vi "DefinePosition.vi"(4 "error in (no error)":errorcluster, 6 "homePosition":i32, 7 "axis in":cluster{"keyHandle":u32, "nodeId":u16}={"keyHandle"=0, "nodeId"=1}) -> (0 "error out":errorcluster, 3 "axis out":cluster{"keyHandle":u32, "nodeId":u16}={"keyHandle"=0, "nodeId"=1})   [LabVIEW 2018]
doc: "<B>DefinePosition</B> writes the new home position to the device. The VI uses the homing method 35 (Actual Position) to define the position."
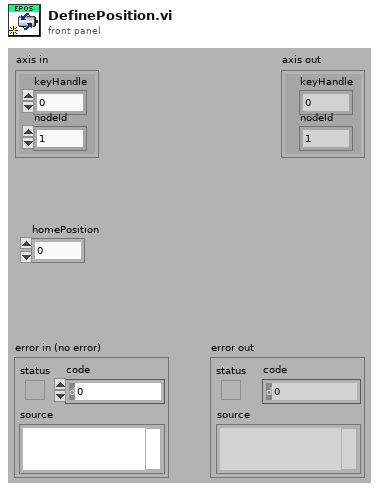
[diagram p1: front panel]
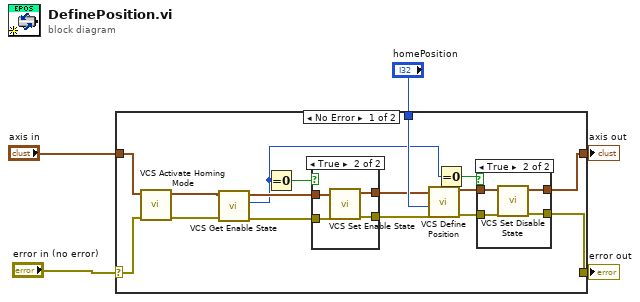
[diagram p0: block diagram]
diagram:
  n1 = case shown="No Error" "error in (no error)" {
    selector: "error in (no error)" -> [w20 w35]
    tunnel: [w8 w35] -> w4
    tunnel: [w7 w34] -> w3
    tunnel: "axis in" -> [w21 w34]
    tunnel: "homePosition" -> [w19 _]
    frame No Error {
      n2 = call "VCS Activate Homing Mode.vi"("error in (no error)"=w20, "axis in"=w21) -> ("error out"=w18:errorcluster, "axis out"=w17:cluster{"keyHandle":u32, "nodeId":u16})  [unwired: 8 in]
      n3 = call "VCS Get Enable State.vi"("error in (no error)"=w18, "axis in"=w17) -> ("error out"=w14:errorcluster, "isEnabled"=w10:i32, "axis out"=w15:cluster{"keyHandle":u32, "nodeId":u16})  [unwired: 7 in]
      n4 = Equal To 0?(x=w10) -> (x = 0?=w16:bool)
      n5 = case shown="True" w16 {
        tunnel: w15 -> [w29 w33]
        tunnel: w14 -> [w28 w32]
        tunnel: [w28 w31] -> w13
        tunnel: [w29 w30] -> w12
        frame False {
        }
        frame True {
          n6 = call "VCS Set Enable State.vi"("error in (no error)"=w32, "axis in"=w33) -> ("error out"=w31:errorcluster, "axis out"=w30:cluster{"keyHandle":u32, "nodeId":u16})  [unwired: 8 in]
        }
      }
      n7 = call "VCS Define Position.vi"("error in (no error)"=w13, "homePosition"=w19, "axis in"=w12) -> ("error out"=w9:errorcluster, "axis out"=w6:cluster{"keyHandle":u32, "nodeId":u16})  [unwired: 7 in]
      n8 = Equal To 0?(x=w10) -> (x = 0?=w11:bool)
      n9 = case shown="True" w11 {
        tunnel: w9 -> [w22 w27]
        tunnel: [w22 w26] -> w8
        tunnel: [w23 w25] -> w7
        tunnel: w6 -> [w23 w24]
        frame False {
        }
        frame True {
          n10 = call "VCS Set Disable State.vi"("error in (no error)"=w27, "axis in"=w24) -> ("error out"=w26:errorcluster, "axis out"=w25:cluster{"keyHandle":u32, "nodeId":u16})  [unwired: 8 in]
        }
      }
    }
    frame Error {
    }
  }
  "error out" <- w4
  "axis out" <- w3
